vi "WriteWorkData.vi"(8 "error in (no error)":errorcluster, 10 "StepData.lvclass":refnum<class "StepData.lvclass">, 11 "AbstractStep in":refnum<class "Move.lvclass">) -> (0 "error out":errorcluster, 3 "AbstractStep out":refnum<class "Move.lvclass">)   [LabVIEW 2014, in "Move.lvclass"]
uses:
  Move.lvclass
  StepData/StepData.lvclass
  Move.lvclass/Move.ctl
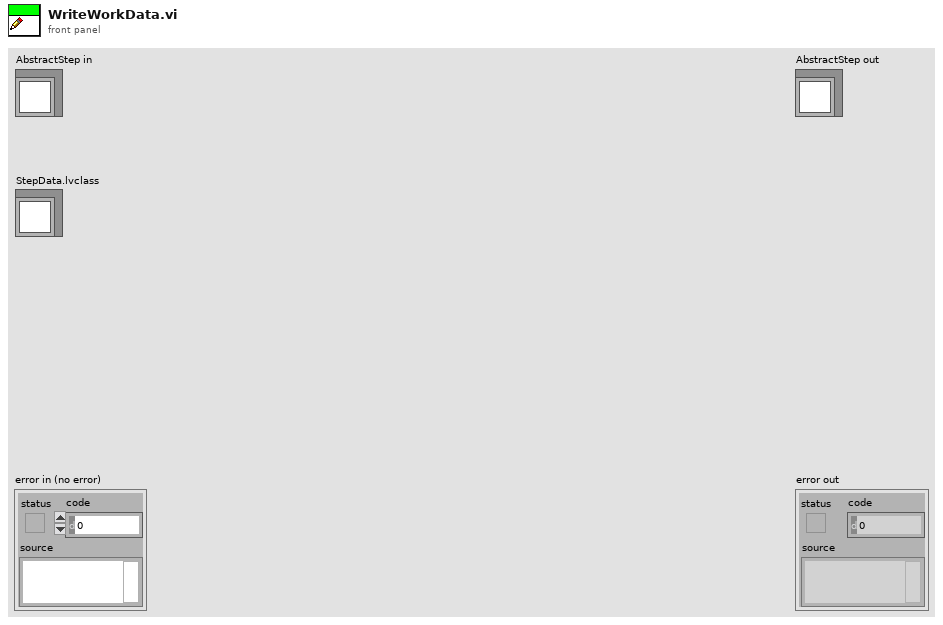
[diagram p1: front panel]
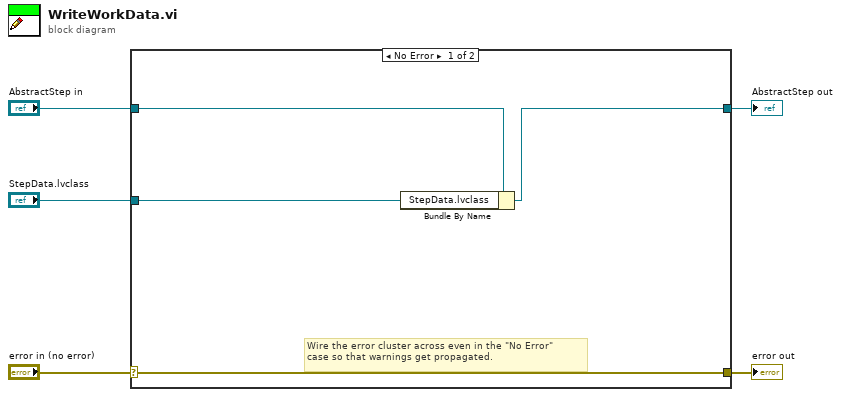
[diagram p0: block diagram]
diagram:
  n1 = case shown="No Error" "error in (no error)" {
    selector: "error in (no error)" -> [w9 w11]
    tunnel: [w9 w11] -> w4
    tunnel: [w6 w10] -> w2
    tunnel: "AbstractStep in" -> [w8 w10]
    tunnel: "StepData.lvclass" -> [w7 _]
    frame No Error {
      # "Wire the error cluster across even in the \"No Error\"\ncase so that warnings get propagated."
      n2 = Bundle By Name(cluster=w8, "StepData.lvclass"=w7) -> (w6:refnum<class "Move.lvclass">)
    }
    frame Error {
    }
  }
  "error out" <- w4
  "AbstractStep out" <- w2
